vi "getClassHierarchyVersions.vi"(8 "error in (no error)":errorcluster, 10 "className":string) -> (0 "error out":errorcluster, 2 "allClassVersionNumbers":u8[][](array[numeric]))   [LabVIEW 2020, in "openg_variant.lvlib" / "Reflection.lvclass"]
doc: "Get the class hierarchy version numbers for the specified class. The first element of the output array is the version number for the input class; the last element is for the top most parent class. Input className can include or exclude the '.lvclass' extension. \n\nGCraftsman JSON Object Serialization Toolkit\nwww.GCraftsman.com\nCopyright (c) 2017, GCraftsman"
uses:
  Reflection.lvclass
  Reflection.lvclass/Reflection.ctl
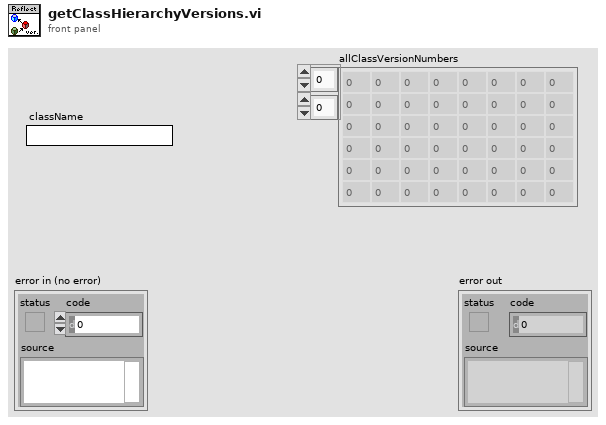
[diagram p1: front panel]
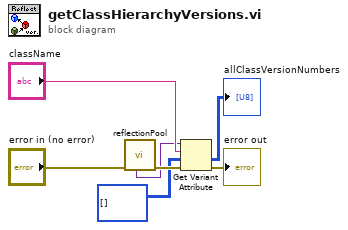
[diagram p0: block diagram]
diagram:
  n1 = call "reflectionPool.vi"("error in (no error)"="error in (no error)") -> ("error out"=w6:errorcluster, "classVersionNumbersLUT"=w1:variant)  [unwired: 5 in, 4 out]
  n2 = Get Variant Attribute(Variant=w1, name="className", default value (empty Variant)=u8[][] [] ("allClassVersionNumbers"), error in=w6) -> (value=→"allClassVersionNumbers":u8[][], error out=→"error out":errorcluster)  [unwired: 2 out]
